vi "Read Control References.vi"(8 "error in":errorcluster, 11 "Instruments in":refnum<class "Instruments.lvclass">) -> (0 "error out":errorcluster, 2 "Control Map":T1[](array[typedef]), 3 "Instruments out":refnum<class "Instruments.lvclass">)   [LabVIEW 2023, in "Instruments.lvlib" / "Instruments.lvclass"]
uses:
  Library/Instruments.lvclass
  C:/Users/Public/Documents/Development/builds/Engine/Engine.lvlibp/Project/Engine.lvclass
  Custom Controls/Control Element.ctl
  builds/Engine/Engine.lvlibp/Accessors/Read VI_Ref.vi
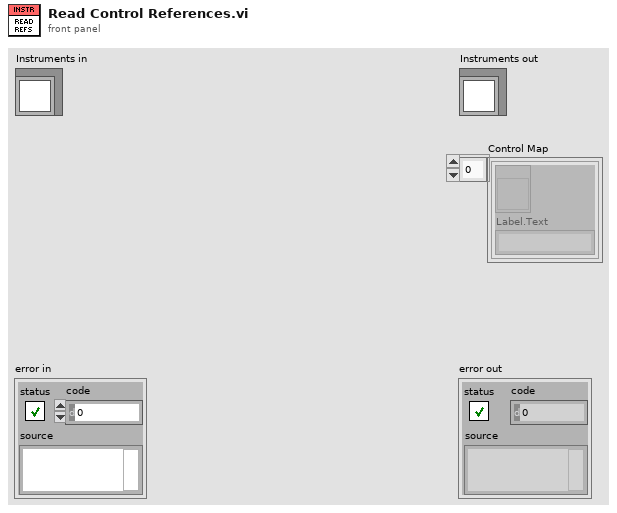
[diagram p1: front panel]
types:
  T1 = typedef "Instruments.lvlib/Instruments.lvclass/Control Element.ctl" = cluster{refnum<vi>, "Label.Text":string}
  T2 = cluster{"Ctl Refnum":refnum<vi>, "Label.Text":string}[]
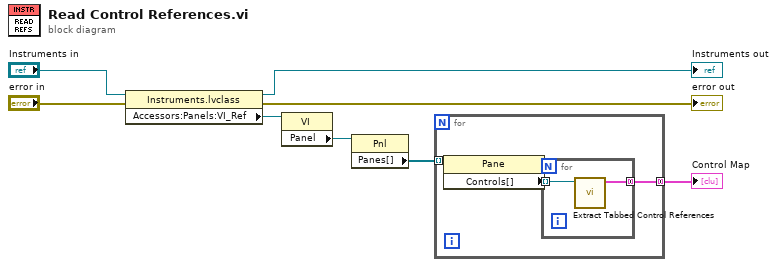
[diagram p0: block diagram]
diagram:
  n1 = property class="Instruments.lvclass"(reference="Instruments in", error in="error in") -> (reference out=→"Instruments out":refnum<class "Instruments.lvclass">, error out=→"error out":errorcluster, "Accessors:Panels:VI_Ref"=w5:refnum<vi>)
  n2 = property class="VI"(reference=w5) -> ("Panel"=w3:refnum<vi>)  [unwired: 1 in, 2 out]
  n3 = property class="Pnl"(reference=w3) -> ("Panes[]"=w2:refnum<vi>[])  [unwired: 1 in, 2 out]
  n4 = for {
    tunnel: w2 -> [w11] mode=indexing
    tunnel: [w9] -> w1 mode=concatenating
    n5 = property class="Pane"(reference=w11) -> ("Controls[]"=w10:refnum<vi>[])  [unwired: 1 in, 2 out]
    n6 = for {
      tunnel: w10 -> [w13] mode=indexing
      tunnel: [w12] -> w9 mode=concatenating
      n7 = call "Extract Tabbed Control References.vi"("Ctl Refnum"=w13) -> ("Control Map"=w12:T2)  [unwired: 10 in]
    }
  }
  "Control Map" <- w1
